vi "TDC_configureFilter.vi"(8 "Error In":errorcluster, 10 "Filter Type":i32(ring)=1 items=["None", "Mute", "Coinc", "Sync", "Invalid"], 11 "Channel":i32) -> (0 "Error Out":errorcluster)   [LabVIEW 2011]
uses:
  tdcbase.dll
panel:
  in  "Channel Mask":i32
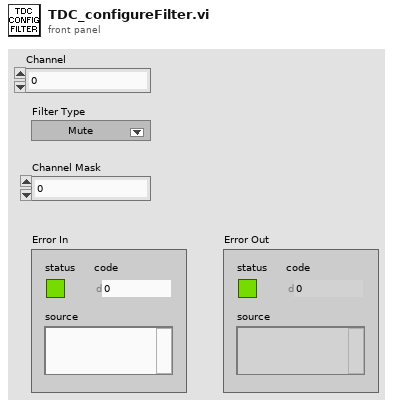
[diagram p1: front panel]
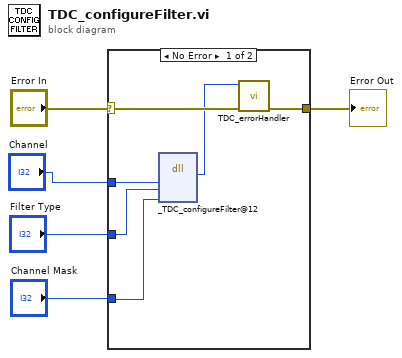
[diagram p0: block diagram]
diagram:
  n1 = case shown="No Error" "Error In" {
    selector: "Error In" -> [w11 w12]
    tunnel: [w10 w12] -> w4
    tunnel: "Channel" -> [w8 _]
    tunnel: "Filter Type" -> [w7 _]
    tunnel: "Channel Mask" -> [w6 _]
    frame No Error {
      n2 = dll-call lib="X:/tdcbase.dll" fn="_TDC_configureFilter@12"("channel"=w8, "filterType"=w7, "channelMask"=w6) -> ("return type"=w9:i32)  [unwired: 6 in, 2 out]
      n3 = call "TDC_errorHandler.vi"("Error In"=w11, "TDC Return Code"=w9) -> ("Error Out"=w10:errorcluster)  [unwired: 9 in]
    }
    frame Error {
    }
  }
  "Error Out" <- w4
